vi "Dashboard Main.vi"() -> ()   [LabVIEW 2016]
uses:
  <vilib>/Utility/miscctls.llb/LVRowAndColumnTypeDef.ctl
  <vilib>/event_ctls.llb/eventvkey.ctl
  <vilib>/Rock Robotics/Network Tables/NT Read Numeric Array.vi
  <vilib>/Rock Robotics/Network Tables/NT Write Boolean.vi
  <vilib>/Rock Robotics/WPI/Dashboard/WPI_DashboardLogging Global.vi
panel:
  out "Background":bool
  in  "Camera Settings Right":T1={"Frame Rate"=30, "Compression"=30, "Size"=1, "DB Camera Config"=FALSE} {"Frame Rate" scale=1.0..30.0; "Compression" scale=100.0..-1.0; "Size" items=["640x480", "320x240", "160x120"]}
  in  "Camera Name Right":string(combo)="No Camera Selection"
  out "Camera Info":cluster{"Mbps LED":bool, "Mbps":dbl, "fps":dbl} {"fps" format="%#.1g"; "Mbps" format="%#.1g"}
  in  "Camera Settings":T1={"Frame Rate"=30, "Compression"=30, "Size"=1, "DB Camera Config"=FALSE} {"Frame Rate" scale=1.0..30.0; "Compression" scale=100.0..-1.0; "Size" items=["640x480", "320x240", "160x120"]}
  in  "TCP":refnum<k5>
  in  "Rec Mode":enum32{"Stop", "Record", "Playback"}(radio)
  out "Robot IP":string
  out "Image Message":string="Timeout in Camera Communications"
  in  "Dashboard Tab":T2(tab)
  in  "GoFast":bool
  in  "Select Auto":string(combo)="Select Autonomous ..."
  out "NT Connection":bool
  out "MotorChart R":cluster{"Numeric":dbl, "Numeric":dbl}(graph)
  out "MotorChart L":cluster{"Numeric":dbl, "Numeric":dbl}(graph)
  out "MotorSliders R":cluster{"MotorSlide1":dbl, "MotorSlide2":dbl} {"MotorSlide2" scale=-1.0..1.0 scale format="%#_2e"; "MotorSlide1" scale=-1.0..1.0 scale format="%#_2e"}
  out "MotorSliders L":cluster{"MotorSlide1":dbl, "MotorSlide2":dbl} {"MotorSlide2" scale=-1.0..1.0 scale format="%#_2e"; "MotorSlide1" scale=-1.0..1.0 scale format="%#_2e"}
  out "Gyro":dbl(knob) scale=0.0..360.0
  out "JS1 Z":dbl(slide) scale=-1.0..1.0 scale format="%#_2e"
  out "JS1 Graph":cluster{"X":dbl, "Y":dbl}[](graph)
  out "JS1 Buttons":T3
  out "JS2 Z":dbl(slide) scale=-1.0..1.0 scale format="%#_2e"
  out "JS2 Graph":cluster{"X":dbl, "Y":dbl}[](graph)
  out "JS2 Buttons":T3
  out "Mode":T4(ring)=enum."Auto Disabled"
  in  "Trim":dbl(slide)=0.5612244897959183 scale=0.0..1.0
  out "Sonar":dbl
  out "Camera Image Right":T5(plugin-control)
  in  "DB/String 9":string
  in  "DB/String 8":string
  in  "DB/String 7":string
  in  "DB/String 6":string
  in  "DB/String 5":string
  in  "DB/String 4":string
  in  "DB/String 3":string
  in  "DB/String 2":string
  in  "DB/String 1":string
  in  "DB/String 0":string
  in  "DB/Slider 0":dbl(slide) scale=0.0..1.0
  in  "DB/Slider 1":dbl(slide) scale=0.0..5.0
  in  "DB/Slider 2":dbl(slide)=11.111111111111112 caption="Autonomous Stop" scale=0.0..50.0
  in  "DB/Slider 3":dbl(slide)=0.6565656565656566 caption="Autonomous Trim" scale=0.0..1.0
  out "DB/LED 3":bool
  out "DB/LED 2":bool
  out "DB/LED 1":bool
  out "DB/LED 0":bool
  in  "DB/Button 3":bool
  in  "DB/Button 2":bool
  in  "DB/Button 1":bool
  in  "DB/Button 0":bool caption="New Name"
  in  "Scaling factor (V/in)":dbl=0.0098
  out "distance":dbl(slide)=125.0 scale=0.0..250.0 scale format="%3d"
  out "Z Acceleration":dbl
  out "Y Acceleration":dbl
  out "X Acceleration":dbl
  in  "Test Slider":dbl(slide) scale=0.0..100.0 scale format="%#_3g"
  in  "On/Off":bool caption="Solenoid"
  in  "Test Name":u16(ring) items=["Select the test to run..."]
  in  "Test Tree":string(tree)
  in  "Motor":cluster{"Value":dbl, "Enable":bool} {"Value" scale=-1.0..1.0 scale format="%#_3g"}
  out "Progress":T6 {"Test Progress" scale=0.0..100.0}
  in  "Rev/Fwd":cluster{"Forward":bool, "Reverse":bool}
  in  "Test Ring":u16(ring) items=["Monochrome", "Color"]
  out "Cmd Status":string
  in  "Execute Command":bool
  in  "Command Params":string[][](table)
  in  "Command Selection":i32(listbox)
  in  "CheckList":i32(listbox)
  out "Tree":string(tree)
  out "Camera Image":T5(plugin-control)
  in  "Camera Name":string(combo)="No Camera Selection"
  # "HW"
  # "HW"
  # "Joysticks"
  # "Drive Motors"
  # "Front"
  # "Right"
  # "Left"
  # "Back"
  # "This tab is a great place for autonomous settings and robot-specific values.\nPlace controls and indicators inside this tab and match name to\nDashboard Variables on robot. You can also delete this comment."
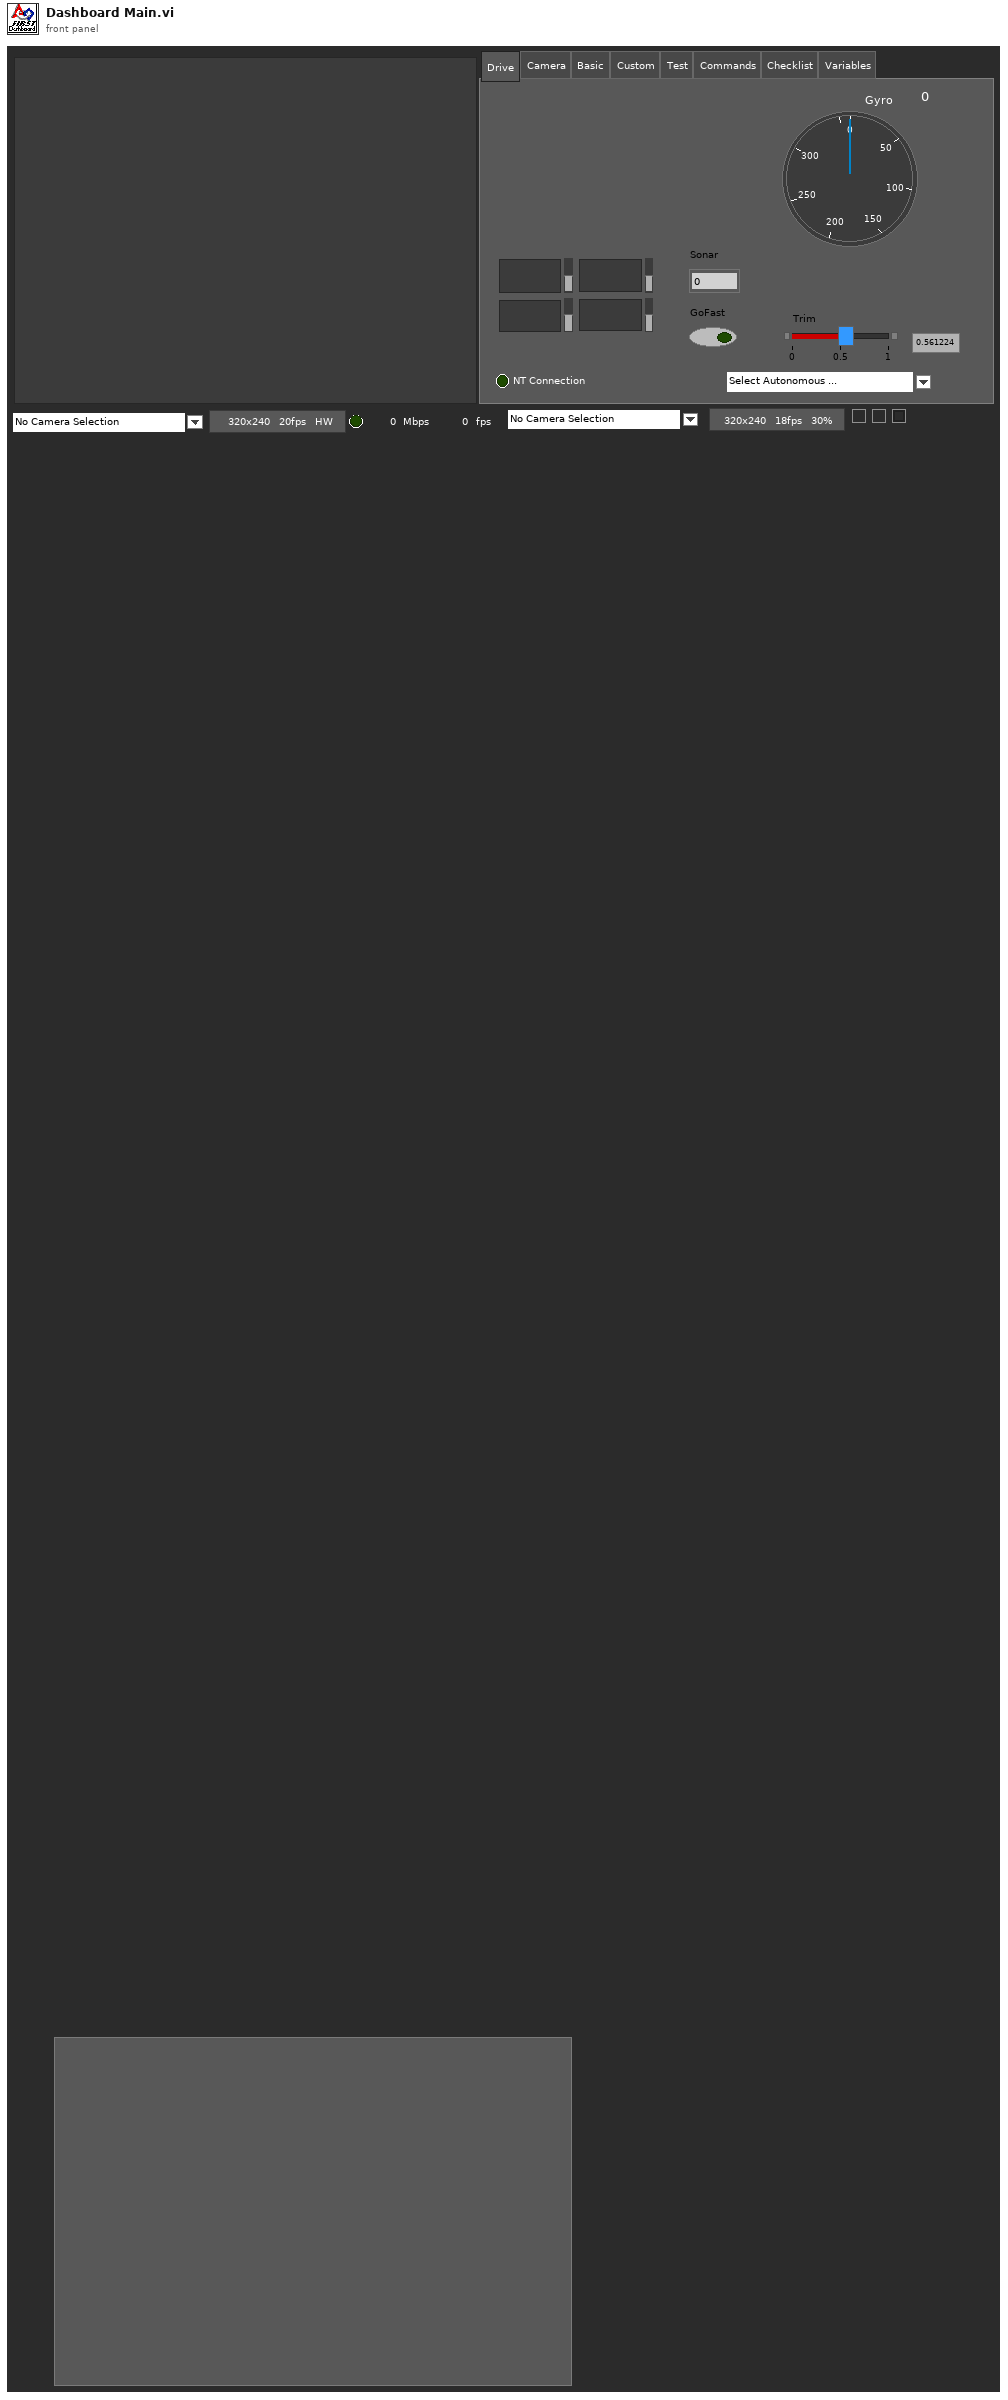
[diagram p1: front panel]
types:
  T1 = cluster{"Frame Rate":i32, "Compression":i32, "Size":u16, "DB Camera Config":bool}
  T2 = enum32{"Drive", "Camera", "Basic", "Custom", "Test", "Commands", "Checklist", "Variables"}
  T3 = cluster{bool, bool, bool, bool, bool, bool, bool, bool, bool, bool, bool, bool}
  T4 = enum8{"Tele-Op Disabled", "Tele-Op Enabled", "Auto Disabled", "Auto Enabled", "Test Disabled", "Test Enabled", "Disconnected", "No Code", "E-Stop"}
  T5 = typedef "IMAQ Image.ctl" = refnum<image>
  T6 = cluster{"Test Progress":u8, "Test Progress Text":string}
  T7 = typedef "Image Type" = u32
  T8 = cluster{"IDs":cluster{"RPC field ID":u16, "Unique ID":u16}, "String":string}
  T9 = enum32{"Drive", "Basic", "Custom", "Test", "Checklist", "Variables"}
  T10 = cluster{"Error Strings":string, "Disable Counts":cluster{u16, u16}, "Rail Faults":cluster{u16, u16, u16}, "Robot IP":string, "DB Mode":u8, "Event Info":cluster{"Name":string, "Type":u8, "Number":u16, "Replay":u8}}
  T11 = cluster{"Storage":cluster{"Disk Free":u64, "RAM Block":u32, "RAM free":u32}, "CPU Utilization":cluster{"CPU % ISR":sgl, "CPU % Time Crit":sgl, "CPU % Timed Str":sgl, "CPU % High":sgl, "CPU % Above":sgl, "CPU % Normal":sgl, "CPU % Low":sgl}, "CAN":cluster{"% Bus Utilization":sgl, "Bus Off Cnt":u32, "TX_FIFO Full Cnt":u32, "Receive Error Cnt":u8, "Transmit Error Cnt":u8}, "HID":cluster{"HID Outputs":u32, "Rumble Low":u16, "Rumble High":u16}[]}
  T12 = cluster{"Status bits":cluster{"Test Mode":bool, "Autonomous":bool, "Enabled":bool, "Code Start":bool, "Brownout":bool, "Reserved 2":bool, "Reserved 3":bool, "E-Stop":bool}, "Code Trace":cluster{"Disabled":bool, "TeleOp":bool, "Auto":bool, "Test":bool}, "Controller Type":enum16{"unknown", "cRIO", "roboRio"}, "Code?":enum16{"unknown", "noCode", "code"}, "Battery V":dbl}
  T13 = cluster{"Control Bits":cluster{"TestMode":bool, "Autonomous":bool, "Enabled":bool, "FMS Present":bool, bool, bool, bool, "E-Stop":bool}, "Team Station ":u8, "Countdown":sgl, "Joystick Values":cluster{"Axes":dbl[], "Buttons":bool[], "POVs":i16[]}[]}
  T14 = cluster{"Axes":dbl[], "Buttons":bool[], "POVs":i16[]}[]
  T15 = cluster{"Axes":dbl[], "Buttons":bool[], "POVs":i16[]}
  T16 = cluster{"Buttons[0]":bool, "Buttons[1]":bool, "Buttons[2]":bool, "Buttons[3]":bool, "Buttons[4]":bool, "Buttons[5]":bool, "Buttons[6]":bool, "Buttons[7]":bool, "Buttons[8]":bool, "Buttons[9]":bool, "Buttons[10]":bool, "Buttons[11]":bool}
  T17 = cluster{"Camera Image":refnum<vi>, "Dashboard Tab":refnum<vi>, "Background":refnum<vi>, "Rec Mode":refnum<vi>, "Test Slider":refnum<vi>, "On/Off ":refnum<vi>, "Test Ring":refnum<vi>, "Rev/Fwd":refnum<vi>, "Test Name":refnum<vi>, "Motor":refnum<vi>, "Progress":refnum<vi>, "CheckList":refnum<vi>, "Tree":refnum<vi>, "Test Tree":refnum<vi>, "Command Params":refnum<vi>, "Command Selection":refnum<vi>, "Execute Command":refnum<vi>, "Cmd Status":refnum<vi>, "Camera Settings":refnum<vi>, "Camera Name":refnum<vi>, "Camera Info":refnum<vi>, "Camera Settings Right":refnum<vi>, "Camera Name Right":refnum<vi>, "Camera Image Right":refnum<vi>}
  T18 = cluster{"Operation":enum16{"Update", "Clear"}, "Color Box":u32}[]
  T19 = typedef "eventvkey.ctl" = enum16{"ASCII", "Enter", "Return", "Shift", "Ctrl", "Alt", "Cmd", "Opt", "Caps", "NumLock", "Clear", "Break", "Up", "Down", "Left", "Right", "Insert", "Delete", "Home", "End", "PageUp", "PageDown", "Escape", "Help", "Pause", "ScrollLock", "F1", "F2", "F3", "F4", "F5", "F6", "F7", "F8", "F9", "F10", "F11", "F12", "F13", "F14", "F15", "F16", "F17", "F18", "F19", "F20", "F21", "F22", "F23", "F24", "Play", "VolumeUp", "VolumeDown", "Mute", "Two Byte Char"}
  T20 = cluster{"Image Size":bool, "Image Type":bool, "Pixel Value":bool, "ROI Information":bool, "Zoom Factor":bool}
  T21 = cluster{"Operation":enum16{"Update", "Clear"}, "Color Box":u32}
  T22 = typedef "LVRowAndColumnTypeDef.ctl" = cluster{"Row":i32, "Column":i32}
  T23 = cluster{"Shift":bool, "Ctrl":bool, "Alt":bool, "Cmd":bool, "Opt":bool}
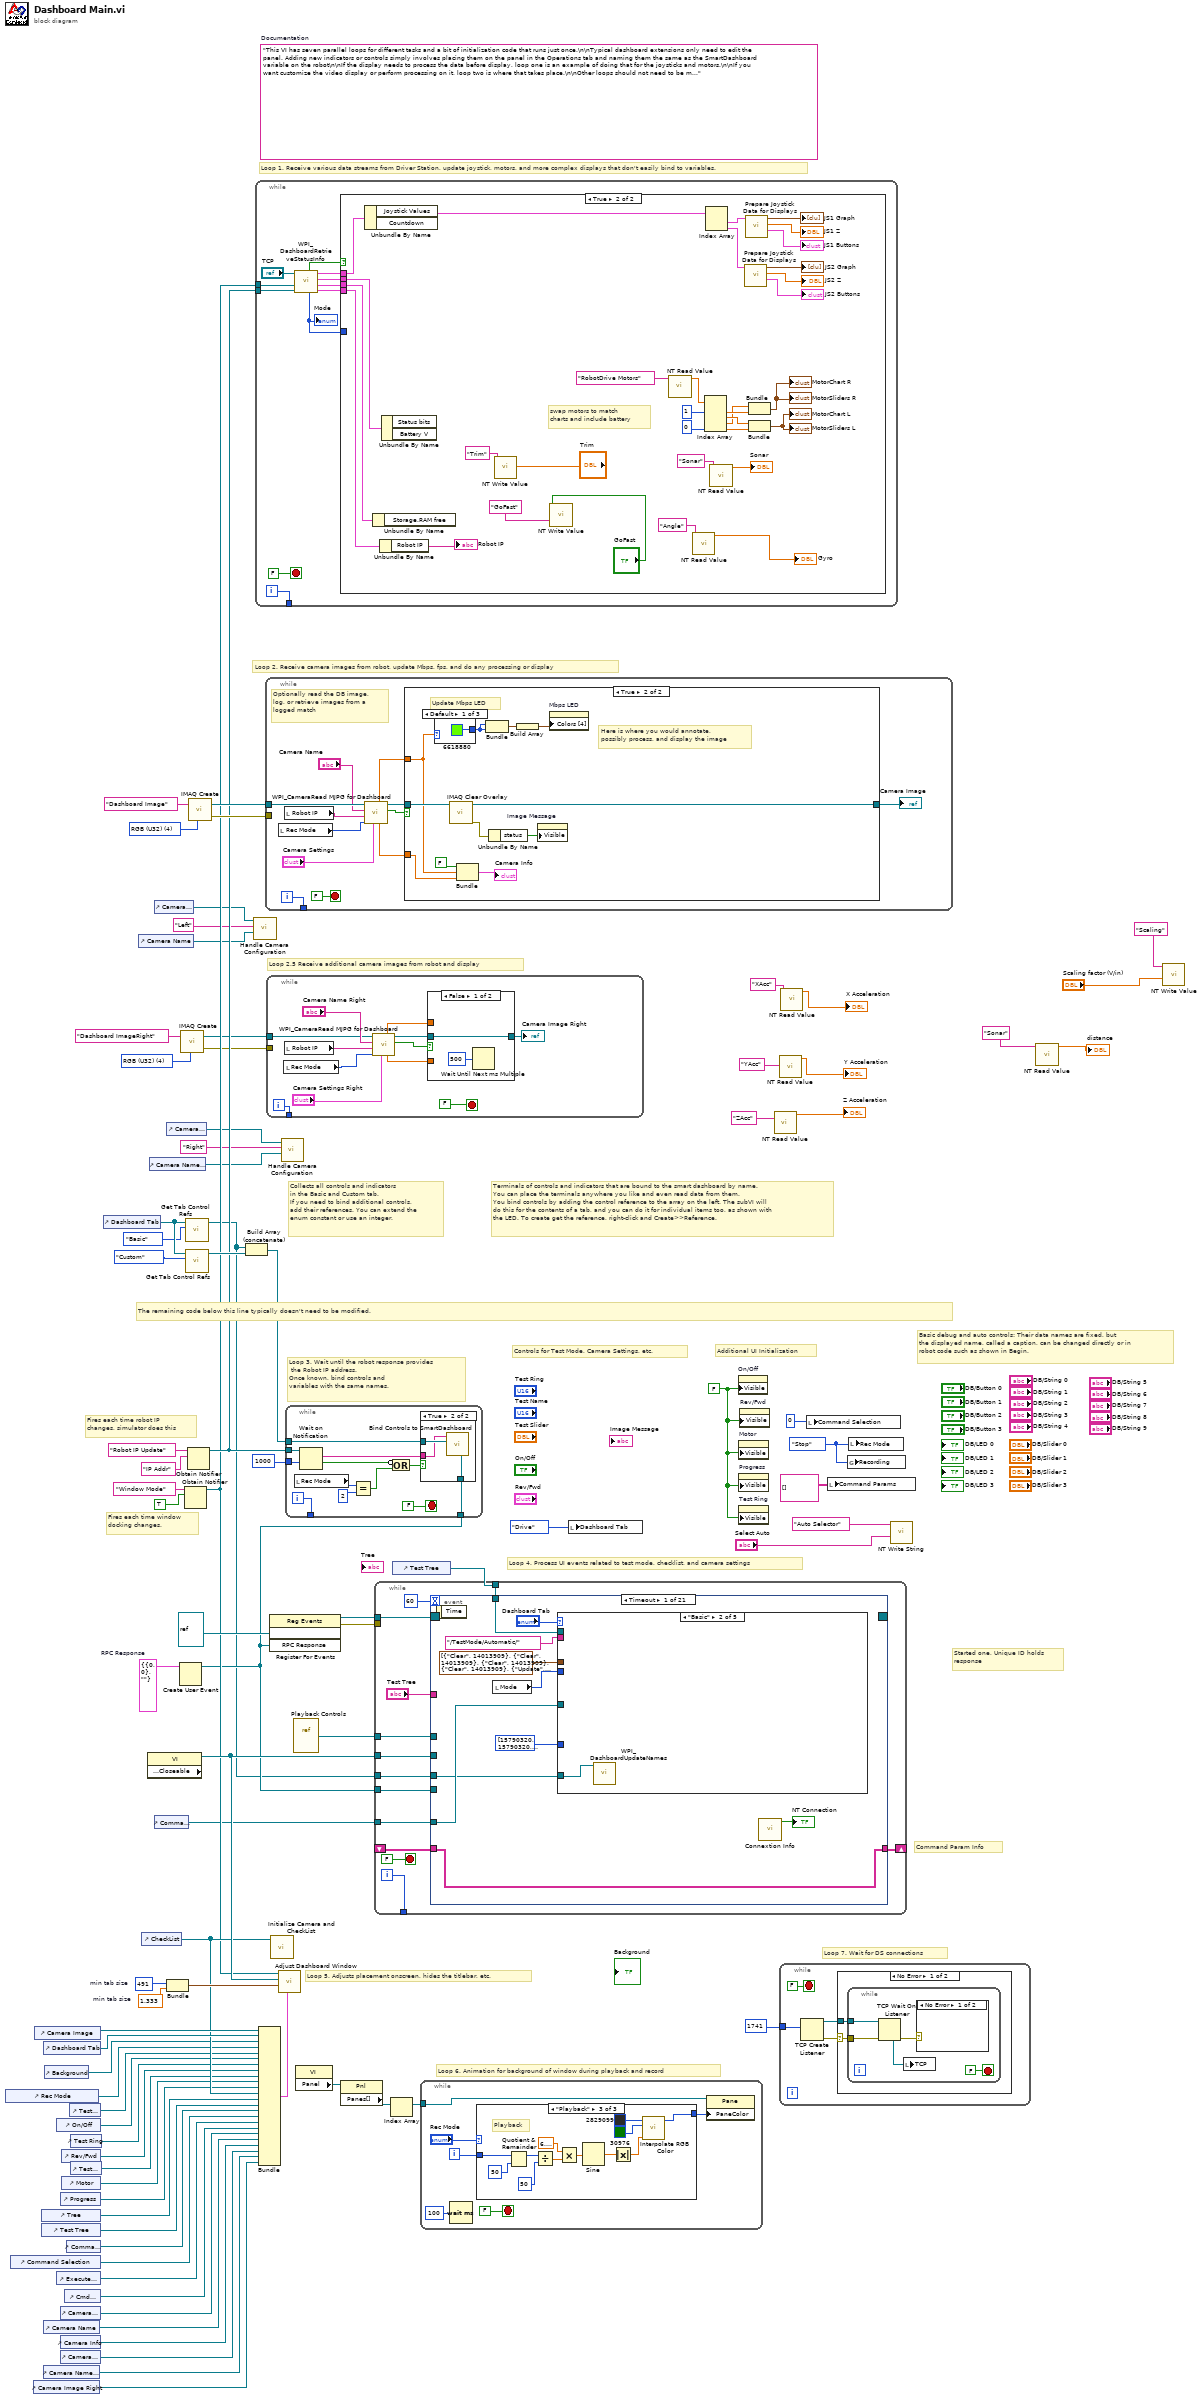
[diagram p0: block diagram]
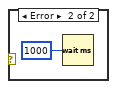
[diagram p3: hidden frame]
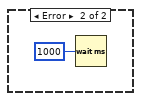
[diagram p4: hidden frame]
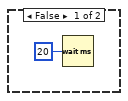
[diagram p5: hidden frame]
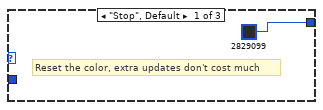
[diagram p6: hidden frame]
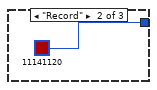
[diagram p7: hidden frame]
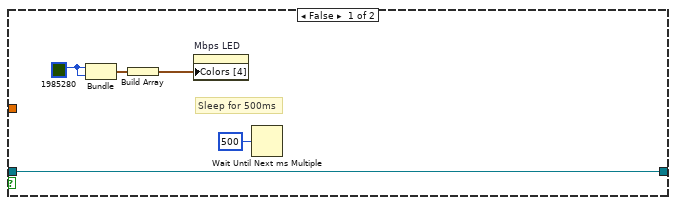
[diagram p9: hidden frame]
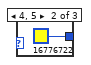
[diagram p10: hidden frame]
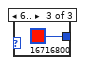
[diagram p11: hidden frame]
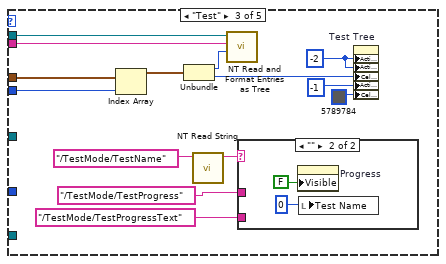
[diagram p13: hidden frame]
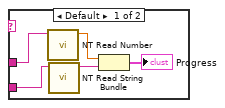
[diagram p14: hidden frame]
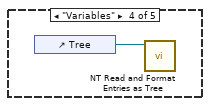
[diagram p15: hidden frame]
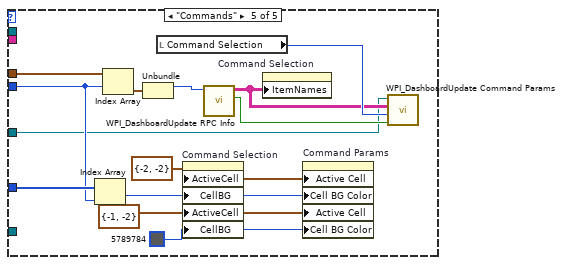
[diagram p16: hidden frame]
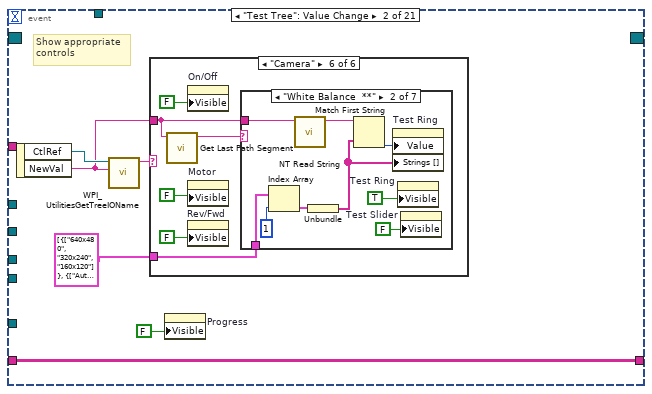
[diagram p17: hidden frame]
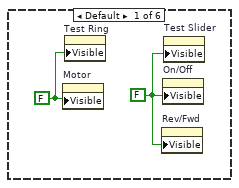
[diagram p18: hidden frame]
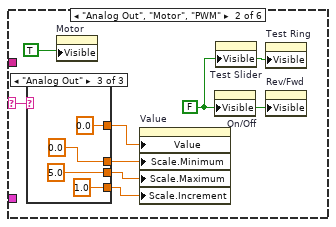
[diagram p19: hidden frame]
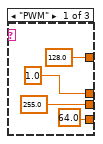
[diagram p20: hidden frame]
diagram:
  w22 = T7 4 items=["Grayscale (U8)", "Grayscale (I16)", "Grayscale (SGL)", "Complex (CSG)", "RGB (U32)", "HSL (U32)", "RGB (U64)"] ("Image Type")
  w38 = T8 {"IDs"={"RPC field ID"=0, "Unique ID"=0}, "String"=""}  # RPC Response
  w61 = 491  # min tab size
  w60 = 1.333  # min tab size
  w68 = enum32{"Stop", "Record", "Playback"}."Stop" ("Rec Mode")
  w45 = FALSE ("Visible")
  (unwired) "This VI has seven parallel loops for different tasks and a bit of initialization code that runs just once.\n\nTypical dashboard extensions only need to edit the panel. Adding new indicators or controls simply involves placing them on the panel in the Operations tab and naming them the same as the SmartDashboard variable on the robot\n\nIf the display needs to process the data before display, loop one is an example of doing that for the joysticks and motors.\n\nIf you want customize the video display or perform processing on it, loop two is where that takes place.\n\nOther loops should not need to be modified. They are pretty standard, and document the task they perform."  # Documentation
  w85 = T7 4 items=["Grayscale (U8)", "Grayscale (I16)", "Grayscale (SGL)", "Complex (CSG)", "RGB (U32)", "HSL (U32)", "RGB (U64)"] ("Image Type")
  # "Loop 2.5 Receive additional camera images from robot and display"
  # "Command Param Info"
  # "Started one, Unique ID holds\nresponse"
  # "Loop 7. Wait for DS connections"
  # "Basic debug and auto controls: Their data names are fixed, but\nthe displayed name, called a caption, can be changed directly or in\nrobot code such as shown in Begin."
  # "Controls for Test Mode, Camera Settings, etc."
  # "Additional UI Initialization"
  # "Loop 6. Animation for background of window during playback and record"
  # "Fires each time robot IP\nchanges, simulator does this"
  # "Fires each time window\ndocking changes."
  # "Collects all controls and indicators\nin the Basic and Custom tab.\nIf you need to bind additional controls,\nadd their references. You can extend the\nenum constant or use an integer."
  # "The remaining code below this line typically doesn't need to be modified."
  # "Loop 4. Process UI events related to test mode, checklist, and camera settings"
  # "Terminals of controls and indicators that are bound to the smart dashboard by name.\nYou can place the terminals anywhere you like and even read data from them.\nYou bind controls by adding the control reference to the array on the left. The subVI will\ndo this for the contents of a tab, and you can do it for individual items too, as shown with\nthe LED. To create get the reference, right-click and Create>>Reference."
  # "Loop 3. Wait until the robot response provides\n the Robot IP address.\nOnce known, bind controls and\nvariables with the same names."
  # "Loop 5. Adjusts placement onscreen, hides the titlebar, etc."
  # "Loop 1. Receive various data streams from Driver Station, update joystick, motors, and more complex displays that don't easily bind to variables."
  # "Loop 2. Receive camera images from robot, update Mbps, fps, and do any processing or display"
  n1 = control-ref of="Rec Mode"() -> (w51:refnum<vi>)
  n2 = control-ref of="Command Selection"() -> (w37:refnum<vi>)
  n3 = control-ref of="Camera Image Right"() -> (w13:refnum<vi>)
  n4 = control-ref of="Camera Image"() -> (w63:refnum<vi>)
  n5 = control-ref of="Tree"() -> (w55:refnum<vi>)
  n6 = control-ref of="Test Tree"() -> (w54:refnum<vi>)
  n7 = control-ref of="Dashboard Tab"() -> (w62:refnum<vi>)
  n8 = control-ref of="Camera Name"() -> (w28:refnum<vi>)
  n9 = control-ref of="Camera Name Right"() -> (w14:refnum<vi>)
  n10 = control-ref of="Background"() -> (w11:refnum<vi>)
  n11 = control-ref of="Execute Command"() -> (w39:refnum<vi>)
  n12 = control-ref of="On/Off"() -> (w49:refnum<vi>)
  n13 = control-ref of="Progress"() -> (w46:refnum<vi>)
  n14 = control-ref of="Camera Settings"() -> (w29:refnum<vi>)
  n15 = control-ref of="Camera Info"() -> (w27:refnum<vi>)
  n16 = control-ref of="Camera Settings Right"() -> (w15:refnum<vi>)
  n17 = control-ref of="Rev/Fwd"() -> (w47:refnum<vi>)
  n18 = control-ref of="Motor"() -> (w52:refnum<vi>)
  n19 = control-ref of="Cmd Status"() -> (w33:refnum<vi>)
  n20 = control-ref of="Command Params"() -> (w40:refnum<vi>)
  n21 = control-ref of="Test Slider"() -> (w50:refnum<vi>)
  n22 = control-ref of="Test Ring"() -> (w48:refnum<vi>)
  n23 = control-ref of="Test Name"() -> (w53:refnum<vi>)
  n24 = control-ref of="Dashboard Tab"() -> (w66:refnum<vi>)
  n25 = control-ref of="Camera Name"() -> (w30:refnum<vi>)
  n26 = control-ref of="CheckList"() -> (w56:refnum<vi>)
  n27 = property class="VI" props=["Front Panel.Closeable"]() -> (reference out=w67:refnum<vi>)  [unwired: 2 in, 2 out]
  n28 = control-ref of="Camera Name Right"() -> (w18:refnum<vi>)
  n29 = control-ref of="Camera Settings"() -> (w31:refnum<vi>)
  n30 = control-ref of="Command Params"() -> (w32:refnum<vi>)
  n31 = control-ref of="Camera Settings Right"() -> (w19:refnum<vi>)
  n32 = Bundle("min tab size"=w61, "min tab size"=w60) -> (w59:cluster{"min tab size":i32, "min tab size":dbl})  [unwired: 1 in]
  n33 = Create User Event(user event datatype=w38) -> (user event=w34:refnum<user-event>)  [unwired: 1 in, 1 out]
  n34 = call "IMAQ Create"("Image Name"="Dashboard ImageRight", "Image Type"=w22) -> ("New Image"=w21:T5, "error out"=w20:errorcluster)  [unwired: 2 in, 1 out]
  n35 = Obtain Notifier(name (unnamed)="Window Mode", notification data type=TRUE) -> (notifier out=w43:refnum<notifier>)  [unwired: 2 in, 2 out]
  n36 = call <vilib>:"Get Tab Control Refs.vi"("Page Index"=T9."Basic" ("Dashboard Tab"), "TabControl in"=w66) -> ("ControlsOnPage"=w26:refnum<vi>[])  [unwired: 9 in]
  n37 = call <vilib>:"Get Tab Control Refs.vi"("Page Index"=T9."Custom" ("Dashboard Tab"), "TabControl in"=w66) -> ("ControlsOnPage"=w65:refnum<vi>[])  [unwired: 9 in]
  n38 = Obtain Notifier(name (unnamed)="Robot IP Update", notification data type="IP Addr" ("name (unnamed)")) -> (notifier out=w44:refnum<notifier>)  [unwired: 2 in, 2 out]
  n39 = call "IMAQ Create"("Image Name"="Dashboard Image", "Image Type"=w85) -> ("New Image"=w83:T5, "error out"=w82:errorcluster)  [unwired: 2 in, 1 out]
  n40 = Build Array (concatenate)(w26, w65) -> (w64:refnum<vi>[])
  n41 = call "Handle Camera Configuration.vi"("CameraNameRef"=w30, "Camera File Name"="Left", "ClusterRef"=w31) -> ()  [unwired: 9 in]
  n42 = while {
    tunnel: [w95] -> _
    tunnel: w44 -> [w89]
    tunnel: w43 -> [w86]
    i -> [w95]
    stop <- FALSE stop-if-true
    n43 = call <vilib>:"WPI_DashboardRetrieveStatusInfo.vi"("Binding Refnum"=w89, "Window Mode Notifier"=w86, "TCP Cnx"="TCP") -> ("Power and Errors"=w90:T10, "Robot Metrics"=w93:T11, "Status Info"=w94:T12, "Control Info"=w91:T13, "Robot Mode"=w88:T4, "Process?"=w92:bool)  [unwired: 3 in]
    "Mode" <- w88
    n44 = case shown="True" w92 {
      tunnel: w94 -> [_ w129]
      tunnel: w93 -> [_ w128]
      tunnel: w91 -> [_ w127]
      tunnel: w90 -> [_ w126]
      tunnel: w88 -> [_ _]
      frame False {
        n45 = Wait (ms)(milliseconds to wait=u32 20) -> ()  [unwired: 1 out]
      }
      frame True {
        # "swap motors to match\ncharts and include battery"
        n46 = Unbundle By Name(w127) -> ("Joystick Values"=w117:T14)  [unwired: 1 out]
        n47 = Unbundle By Name(w128) -> ()  [unwired: 1 out]
        n48 = Unbundle By Name(w126) -> ("Robot IP"=→"Robot IP":string)
        n49 = Unbundle By Name(w129) -> ()  [unwired: 2 out]
        n50 = call-poly <vilib>:"NT Write Value.vi"("Numeric"="Trim", "Name"="Trim") -> ()  [unwired: 9 in, 1 out]
        n51 = call-poly <vilib>:"NT Write Value.vi"("Boolean"="GoFast", "Name"="GoFast") -> ()  [unwired: 9 in, 1 out]
        n52 = call-poly <vilib>:"NT Read Value.vi"("Name"="RobotDrive Motors") -> ("Numeric Array"=w107:dbl[])  [unwired: 9 in, 1 out]
        n53 = call-poly <vilib>:"NT Read Value.vi"("Name"="Angle") -> ("Numeric"=→"Gyro":dbl)  [unwired: 9 in, 1 out]
        n54 = Index Array(array=w107, index #1=1, index #4=0) -> (element #1=w121:dbl, element #2=w122:dbl, element #3=w120:dbl, element #4=w125:dbl)  [unwired: 2 in]
        n55 = Index Array(array=w117) -> (element #1=w116:T15, element #2=w112:T15)  [unwired: 2 in]
        n56 = call-poly <vilib>:"NT Read Value.vi"("Name"="Sonar") -> ("Numeric"=→"Sonar":dbl)  [unwired: 9 in, 1 out]
        n57 = call "Prepare Joystick Data for Displays.vi"("Joystick Values"=w112) -> ("Buttons"=→"JS2 Buttons":T16, "Z Axis"=→"JS2 Z":dbl, "Cartesian Data"=→"JS2 Graph":cluster{"X axis":dbl, "X axis":dbl}[])  [unwired: 8 in]
        n58 = call "Prepare Joystick Data for Displays.vi"("Joystick Values"=w116) -> ("Buttons"=→"JS1 Buttons":T16, "Z Axis"=→"JS1 Z":dbl, "Cartesian Data"=→"JS1 Graph":cluster{"X axis":dbl, "X axis":dbl}[])  [unwired: 8 in]
        n59 = Bundle("Numeric"=w120, "Numeric"=w121) -> (→"MotorChart R" →"MotorSliders R":cluster{"Numeric":dbl, "Numeric":dbl})  [unwired: 1 in]
        n60 = Bundle("Numeric"=w122, "Numeric"=w125) -> (→"MotorChart L" →"MotorSliders L":cluster{"Numeric":dbl, "Numeric":dbl})  [unwired: 1 in]
      }
    }
  }
  n61 = Bundle("Camera Image"=w63, "Dashboard Tab"=w62, "Background"=w11, "Rec Mode"=w51, "Test Slider"=w50, "On/Off"=w49, "Test Ring"=w48, "Rev/Fwd"=w47, "Test Name"=w53, "Motor"=w52, "Progress"=w46, "CheckList"=w56, "Tree"=w55, "Test Tree"=w54, "Command Params"=w40, "Command Selection"=w37, "Execute Command"=w39, "Cmd Status"=w33, "Camera Settings"=w29, "Camera Name"=w28, "Camera Info"=w27, "Camera Settings Right"=w15, "Camera Name Right"=w14, "Camera Image Right"=w13) -> (w12:T17)  [unwired: 1 in]
  n62 = while {
    tunnel: w83 -> [w139]
    tunnel: w82 -> [_]
    tunnel: [w140] -> _
    i -> [w140]
    stop <- FALSE stop-if-true
    # "Optionally read the DB image,\nlog, or retrieve images from a\nlogged match"
    n63 = local read "Rec Mode"() -> (w135:enum32{"Stop", "Record", "Playback"})
    n64 = local read "Robot IP"() -> (w134:string)
    n65 = call <vilib>:"WPI_CameraRead MJPG for Dashboard.vi"("Camera Settings"="Camera Settings", "Rec Mode"=w135, "Robot IP"=w134, "Camera Name"="Camera Name", "Refnum in"=w139) -> ("Active"=w137:bool, "Refnum out"=w138:T5, "FPS"=w136:dbl, "Bandwidth (Mbps)"=w133:dbl)  [unwired: 3 in]
    n66 = case shown="True" w137 {
      tunnel: w138 -> [w142 w153]
      tunnel: w133 -> [_ w150]
      tunnel: w136 -> [_ w151]
      tunnel: [w142 w147] -> w130
      frame False {
        w144 = u32 1985280 ("Color Box")
        # "Sleep for 500ms"
        n67 = Bundle("Color Box"=w144, "Color Box"=w144) -> (w145:cluster{"Color Box":u32, "Color Box":u32})  [unwired: 1 out]
        n68 = Build Array(w145) -> (w143:cluster{"Color Box":u32, "Color Box":u32}[])
        n69 = property on="Mbps LED" class="Bool (strict)"("Colors [4]"=w143) -> ()  [unwired: 2 in, 2 out]
        n70 = Wait Until Next ms Multiple(millisecond multiple=u32 500) -> ()  [unwired: 1 out]
      }
      frame True {
        # "Here is where you would annotate,\npossibly process, and display the image"
        # "Update Mbps LED"
        n71 = case shown="Default" w150 {
          tunnel: [u32 6618880 ("Color Box") u32 16776722 ("Color Box") u32 16716800 ("Color Box")] -> w154
          frame Default {
          }
          frame 4, 5 {
          }
          frame 6.. {
          }
        }
        n72 = call "IMAQ Clear Overlay"("Image"=w153) -> ("error out"=w156:errorcluster, "Image Out"=w147:T5)  [unwired: 2 in, 7 out]
        n73 = Bundle(FALSE, "Bandwidth (Mbps)"=w150, "FPS"=w151) -> (→"Camera Info":cluster{bool, "Bandwidth (Mbps)":dbl, "FPS":dbl})  [unwired: 1 in]
        n74 = Bundle("Color Box"=w154, "Color Box"=w154) -> (w155:cluster{"Color Box":u32, "Color Box":u32})  [unwired: 1 out]
        n75 = Unbundle By Name(w156) -> ("status"=w157:bool)
        n76 = Build Array(w155) -> (w152:cluster{"Color Box":u32, "Color Box":u32}[])
        n77 = property on="Image Message" class="Str"("Visible"=w157) -> ()  [unwired: 2 in, 2 out]
        n78 = property on="Mbps LED" class="Bool (strict)"("Colors [4]"=w152) -> ()  [unwired: 2 in, 2 out]
      }
    }
    "Camera Image" <- w130
  }
  n79 = while {
    tunnel: w21 -> [w171]
    tunnel: w20 -> [_]
    tunnel: [w165] -> _
    i -> [w165]
    stop <- FALSE stop-if-true
    n80 = local read "Rec Mode"() -> (w169:enum32{"Stop", "Record", "Playback"})
    n81 = local read "Robot IP"() -> (w170:string)
    n82 = call <vilib>:"WPI_CameraRead MJPG for Dashboard.vi"("Camera Settings"="Camera Settings Right", "Rec Mode"=w169, "Robot IP"=w170, "Camera Name"="Camera Name Right", "Refnum in"=w171) -> ("Active"=w164:bool, "Refnum out"=w167:T5, "FPS"=w162:dbl, "Bandwidth (Mbps)"=w163:dbl)  [unwired: 3 in]
    n83 = case shown="False" w164 {
      tunnel: w167 -> [w173 w175]
      tunnel: w163 -> [_ _]
      tunnel: w162 -> [_ _]
      tunnel: [w173 w175] -> w161
      frame False {
        n84 = Wait Until Next ms Multiple(millisecond multiple=u32 500) -> ()  [unwired: 1 out]
      }
      frame True {
      }
    }
    "Camera Image Right" <- w161
  }
  n85 = register-events(refnum<vi> refnum, w34) -> (reference out=w72:refnum<event-registration>, error out=w71:errorcluster)  [unwired: 2 in]
  n86 = call "Initialize Camera and CheckList.vi"("ListBox in"=w56) -> ()  [unwired: 11 in]
  n87 = call "Adjust Dashboard Window.vi"("Sizing Refnums"=w12, "Size Constraints"=w59, "VI"=w67, "WIn Mode"=w43) -> ()  [unwired: 8 in]
  n88 = call "Handle Camera Configuration.vi"("CameraNameRef"=w18, "Camera File Name"="Right", "ClusterRef"=w19) -> ()  [unwired: 9 in]
  n89 = while {
    tunnel: w64 -> [w187]
    tunnel: w44 -> [w185]
    tunnel: [w183] -> _
    tunnel: u32 1000 ("milliseconds to wait") -> [w182]
    tunnel: w34 -> [w176]
    i -> [w183]
    stop <- FALSE stop-if-true
    n90 = local read "Rec Mode"() -> (w178:enum32{"Stop", "Record", "Playback"})
    n91 = Wait on Notification(notifier=w185, timeout in ms (-1)=w182) -> (notification=w184:string, timed out?=w180:bool)  [unwired: 2 in, 2 out]
    n92 = Equal?(x=w178, y=u16 2 ("Rec Mode")) -> (x = y?=w179:bool)
    n93 = Compound Arithmetic op=OR(invert w180, w179) -> (w181:bool)
    n94 = case shown="True" w181 {
      tunnel: w187 -> [_ w190]
      tunnel: w184 -> [_ w189]
      tunnel: w176 -> [_ w188]
      frame False {
      }
      frame True {
        n95 = call <vilib>:"Bind Controls to SmartDashboard.vi"("RPC ref"=w188, "Bound Control Refs"=w190, "Server IP Address"=w189) -> ()  [unwired: 9 in]
      }
    }
  }
  n96 = vi-ref "Playback Controls.vi"() -> (w73:refnum<vi>)
  n97 = property class="VI"() -> ("Panel"=w75:refnum<vi>)  [unwired: 2 in, 2 out]
  n98 = property class="Pnl"(reference=w75) -> ("Panes[]"=w76:refnum<vi>[])  [unwired: 1 in, 2 out]
  n99 = Index Array(array=w76) -> (element=w74:refnum<vi>)  [unwired: 1 in]
  n100 = control-ref of="Test Tree"() -> (w77:refnum<vi>)
  n101 = while {
    tunnel: [w200] -> _
    tunnel: w77 -> [w199]
    tunnel: w73 -> [w198]
    tunnel: w72 -> [w197]
    tunnel: w71 -> [_]
    tunnel: w67 -> [w196]
    tunnel: w34 -> [w195]
    tunnel: w32 -> [w194]
    shift-right: [w193] -> _
    shift-left: _ -> [w192]
    tunnel: w26 -> [w191]
    i -> [w200]
    stop <- FALSE stop-if-true
    n102 = event shown="[0] Timeout" {
      selector: w197 -> [_ _ _ _ _ _ _ _ _ _ _ _ _ _ _ _ _ _ _ _ _]
      dyn-events: [_ _ _ _ _ _ _ _ _ _ _ _ _ _ _ _ w456 _ _ _ _] -> _
      timeout: u32 60 ("milliseconds to wait") -> [_ _ _ _ _ _ _ _ _ _ _ _ _ _ _ _ _ _ _ _ _]
      tunnel: w199 -> [w212 _ _ _ _ _ _ _ _ _ _ _ _ _ _ _ _ _ _ _ _]
      tunnel: "Test Tree" -> [_ _ _ _ _ _ _ _ _ _ _ w423 w431 w433 w437 w445 _ _ _ _ _]
      tunnel: w198 -> [_ _ _ _ _ _ _ _ _ _ _ _ _ _ _ _ w458 _ w476 _ _]
      tunnel: w196 -> [_ _ _ _ _ _ _ _ _ _ _ _ _ _ _ _ w454 _ _ _ _]
      tunnel: w195 -> [_ _ _ _ _ _ _ _ _ _ _ _ _ _ _ _ w450 _ _ _ _]
      tunnel: w194 -> [w207 _ _ _ _ _ w374 _ _ _ _ _ _ _ _ _ _ _ _ _ _]
      tunnel: [w206 w251 w353 w358 w367 w371 w372 w381 w391 w398 w410 w422 w429 w432 w436 w444 w449 w471 w473 w477 w488] -> w193
      tunnel: w192 -> [w206 w251 w353 w358 w367 w371 w372 _ _ w398 w410 w422 w429 w432 w436 w444 w449 w471 w473 w477 w488]
      tunnel: w191 -> [w204 _ _ _ _ _ _ _ _ _ _ _ _ _ _ _ _ _ _ _ _]
      event Timeout {
        n103 = event-data() -> ()  [unwired: 1 in, 1 out]
        n104 = local read "Mode"() -> (w209:T4)
        n105 = case shown="\"Basic\"" "Dashboard Tab" {
          tunnel: w212 -> [_ _ w228 _ _]
          tunnel: "/TestMode/Automatic/" ("Name Pattern") -> [_ _ w227 _ _]
          tunnel: T18 [{"Operation"=enum."Clear", "Color Box"=14013909}, {"Operation"=enum."Clear", "Color Box"=14013909}, {"Operation"=enum."Clear", "Color Box"=14013909}, {"Operation"=enum."Clear", "Color Box"=14013909}, {"Operation"=enum."Update", "Color Box"=14013909}, {"Operation"=enum."Update", "Color Box"=16777215}, {"Operation"=enum."Clear", "Color Box"=14013909}, {"Operation"=enum."Clear", "Color Box"=14013909}, {"Operation"=enum."Clear", "Color Box"=14013909}] -> [_ _ w220 _ w244]
          tunnel: w209 -> [_ _ w219 _ w243]
          tunnel: u32[] [15790320, 15790320, 15790320, 15790320, 16777215, 16777215, 15790320, 15790320, 15790320] -> [_ _ _ _ w249]
          tunnel: w207 -> [_ _ _ _ w237]
          tunnel: w204 -> [_ w214 _ _ _]
          frame "Custom", Default {
          }
          frame "Basic" {
            n106 = call <vilib>:"WPI_DashboardUpdateNames.vi"("Controls on Tab"=w214) -> ()  [unwired: 11 in]
          }
          frame "Test" {
            w226 = -2 ("Active Item:Row Number")
            n107 = Index Array(array=w220, index=w219) -> (element=w221:T21)
            n108 = Unbundle(w221) -> ("Operation"=w222:enum16{"Update", "Clear"}, "Color Box"=w223:u32)
            n109 = call <vilib>:"NT Read String.vi"("Name"="/TestMode/TestName") -> ("String"=w217:string)  [unwired: 9 in, 1 out]
            n110 = call <vilib>:"NT Read and Format Entries as Tree.vi"("Operation"=w222, "Name Pattern"=w227, "Tree Refnum"=w228) -> ()  [unwired: 7 in, 2 out]
            n111 = case shown="\"\"" w217 {
              tunnel: "/TestMode/TestProgress" ("Name") -> [w230 _]
              tunnel: "/TestMode/TestProgressText" ("Name") -> [w229 _]
              frame Default {
                n112 = call <vilib>:"NT Read Number.vi"("Name"=w230) -> ("Numeric"=w231:dbl)  [unwired: 9 in, 1 out]
                n113 = call <vilib>:"NT Read String.vi"("Name"=w229) -> ("String"=w232:string)  [unwired: 9 in, 1 out]
                n114 = Bundle("Numeric"=w231, "String"=w232) -> (→"Progress":cluster{"Numeric":dbl, "String":string})  [unwired: 1 in]
              }
              frame "" {
                n115 = property on="Progress" class="Clust (strict)"("Visible"=FALSE) -> ()  [unwired: 2 in, 2 out]
                n116 = local write "Test Name"(u16 0) -> ()
              }
            }
            n117 = property on="Test Tree" class="Tree (strict)"("Active Item Row Number"=w226, "ActiveColNum"=w226, "CellBG"=w223, "Active Item Row Number"=-1 ("Active Item:Row Number"), "CellBG"=u32 5789784 ("Color Box")) -> ()  [unwired: 2 in, 2 out]
          }
          frame "Variables" {
            n118 = control-ref of="Tree"() -> (w236:refnum<vi>)
            n119 = call <vilib>:"NT Read and Format Entries as Tree.vi"("Tree Refnum"=w236) -> ()  [unwired: 9 in, 2 out]
          }
          frame "Commands" {
            w245 = u32 5789784 ("Color Box")
            w246 = T22 {"Row"=-1, "Column"=-2} ("Active Cell:Active Cell")
            w248 = T22 {"Row"=-2, "Column"=-2} ("Active Cell:Active Cell")
            n120 = Index Array(array=w249, index=w243) -> (element=w247:u32)
            n121 = Index Array(array=w244, index=w243) -> (element=w242:T21)
            n122 = Unbundle(w242) -> ("Operation"=w241:enum16{"Update", "Clear"})  [unwired: 1 out]
            n123 = local read "Command Selection"() -> (w240:i32)
            n124 = property on="Command Selection" class="MCListbox (strict)"("ActiveCell"=w248, "CellBG"=w247, "ActiveCell"=w246, "CellBG"=w245) -> ()  [unwired: 2 in, 2 out]
            n125 = call <vilib>:"WPI_DashboardUpdate RPC Info.vi"("Operation"=w241) -> ("update"=w239:bool, "commands"=w238:string[][])  [unwired: 9 in]
            n126 = property on="Command Selection" class="MCListbox (strict)"("ItemNames"=w238) -> ()  [unwired: 2 in, 2 out]
            n127 = property on="Command Params" class="Tbl (strict)"("Active Cell"=w248, "Cell BG Color"=w247, "Active Cell"=w246, "Cell BG Color"=w245) -> ()  [unwired: 2 in, 2 out]
            n128 = call <vilib>:"WPI_DashboardUpdate Command Params.vi"("Update"=w239, "NewVal"=w240, "Commands"=w238, "Param Tbl"=w237) -> ()  [unwired: 7 in, 1 out]
          }
        }
        n129 = call <vilib>:"Connextion Info.vi"() -> ("Connected"=→"NT Connection":bool)  [unwired: 10 in, 1 out]
      }
      event "Test Tree": Value Change {
        # "Show appropriate\ncontrols"
        n130 = event-data() -> ("CtlRef"=w254:refnum<vi>, "NewVal"=w252:string)  [unwired: 1 in]
        n131 = call <vilib>:"WPI_UtilitiesGetTreeIOName.vi"("NewVal"=w252, "TreeControl in"=w254) -> ("I/O Name"=w255:string)  [unwired: 9 in]
        n132 = case shown="\"Camera\"" w255 {
          selector: w255 -> [_ w262 _ w284 w293 _]
          tunnel: w252 -> [_ _ w281 w283 _ w300]
          tunnel: cluster{string[]}[] [{["640x480", "320x240", "160x120"]}, {["Auto", "Fixed indoor", "Fixed outdoor 1", "Fixed outdoor 2", "Fixed fluorescent 1", "Fixed fluorescent 2", "Hold current"]}, {["Auto", "Flicker-free 50 Hz", "Flicker-free 60 Hz", "Hold current"]}, {["None", "Prioritize frame rate", "Prioritize image quality"]}, {["Monochrome", "Color"]}] -> [_ _ _ _ _ w299]
          frame Default {
            w257 = FALSE ("Visible")
            w256 = FALSE ("Visible")
            n133 = property on="Motor" class="Clust (strict)"("Visible"=w256) -> ()  [unwired: 2 in, 2 out]
            n134 = property on="Test Ring" class="Ring (strict)"("Visible"=w256) -> ()  [unwired: 2 in, 2 out]
            n135 = property on="Rev/Fwd" class="Clust (strict)"("Visible"=w257) -> ()  [unwired: 2 in, 2 out]
            n136 = property on="On/Off" class="Bool (strict)"("Visible"=w257) -> ()  [unwired: 2 in, 2 out]
            n137 = property on="Test Slider" class="Slide (strict)"("Visible"=w257) -> ()  [unwired: 2 in, 2 out]
          }
          frame "Analog Out", "Motor", "PWM" {
            w263 = FALSE ("Visible")
            n138 = case shown="\"Analog Out\"" w262 {
              tunnel: [1.0 ("Value") -1.0 ("Value") 0.0 ("Value")] -> w261
              tunnel: [255.0 ("Value") 1.0 ("Value") 5.0 ("Value")] -> w260
              tunnel: [128.0 ("Value") 0.0 ("Value") 0.0 ("Value")] -> w259
              tunnel: [64.0 ("Value") 0.5 ("Value") 1.0 ("Value")] -> w258
              frame "PWM" {
              }
              frame "Motor", Default {
              }
              frame "Analog Out" {
              }
            }
            n139 = property on="Motor" class="Clust (strict)"("Visible"=TRUE) -> ()  [unwired: 2 in, 2 out]
            n140 = property on="Value" class="Slide (strict)"("Value"=w259, "Scale.Minimum"=w261, "Scale.Maximum"=w260, "Scale.Increment"=w258) -> ()  [unwired: 2 in, 2 out]
            n141 = property on="On/Off" class="Bool (strict)"("Visible"=w263) -> ()  [unwired: 2 in, 2 out]
            n142 = property on="Test Slider" class="Slide (strict)"("Visible"=w263) -> ()  [unwired: 2 in, 2 out]
            n143 = property on="Test Ring" class="Ring (strict)"("Visible"=w263) -> ()  [unwired: 2 in, 2 out]
            n144 = property on="Rev/Fwd" class="Clust (strict)"("Visible"=w263) -> ()  [unwired: 2 in, 2 out]
          }
          frame "Servo" {
            w279 = FALSE ("Visible")
            n145 = call <vilib>:"NT Read Number.vi"("Name"=w281) -> ("Numeric"=w280:dbl)  [unwired: 9 in, 1 out]
            n146 = property on="Test Slider" class="Slide (strict)"("Visible"=TRUE, "Scale.Maximum"=170.0 ("Scale.Range:Maximum")) -> ()  [unwired: 2 in, 2 out]
            n147 = local write "Test Slider"(w280) -> ()
            n148 = property on="Motor" class="Clust (strict)"("Visible"=w279) -> ()  [unwired: 2 in, 2 out]
            n149 = property on="Rev/Fwd" class="Clust (strict)"("Visible"=w279) -> ()  [unwired: 2 in, 2 out]
            n150 = property on="On/Off" class="Bool (strict)"("Visible"=w279) -> ()  [unwired: 2 in, 2 out]
            n151 = property on="Test Ring" class="Ring (strict)"("Visible"=w279) -> ()  [unwired: 2 in, 2 out]
          }
          frame "Relay", "Solenoid" {
            w282 = FALSE ("Visible")
            n152 = property on="Motor" class="Clust (strict)"("Visible"=w282) -> ()  [unwired: 2 in, 2 out]
            n153 = property on="Test Slider" class="Slide (strict)"("Visible"=w282) -> ()  [unwired: 2 in, 2 out]
            n154 = Search and Replace String(input string=w283, search string="/Value  **", replace string="/Direction") -> (result string=w289:string)  [unwired: 5 in, 3 out]
            n155 = property on="Test Ring" class="Ring (strict)"("Visible"=w282) -> ()  [unwired: 2 in, 2 out]
            n156 = call <vilib>:"NT Read String.vi"("Name"=w289) -> ("String"=w287:string)  [unwired: 9 in, 1 out]
            n157 = Equal?(x="Both directions", y=w287) -> (x = y?=w285:bool)
            n158 = Not(x=w285) -> (.not. x?=w286:bool)
            n159 = property on="Rev/Fwd" class="Clust (strict)"("Visible"=w285) -> ()  [unwired: 2 in, 2 out]
            n160 = property on="On/Off" class="Bool (strict)"("Visible"=w286, "Caption.Text"=w284) -> ()  [unwired: 2 in, 2 out]
          }
          frame "Compressor", "Digital Out" {
            w292 = FALSE ("Visible")
            # "Get direction and finish"
            n161 = property on="Motor" class="Clust (strict)"("Visible"=w292) -> ()  [unwired: 2 in, 2 out]
            n162 = property on="Test Slider" class="Slide (strict)"("Visible"=w292) -> ()  [unwired: 2 in, 2 out]
            n163 = property on="Test Ring" class="Ring (strict)"("Visible"=w292) -> ()  [unwired: 2 in, 2 out]
            n164 = property on="On/Off" class="Bool (strict)"("Visible"=TRUE, "Caption.Text"=w293) -> ()  [unwired: 2 in, 2 out]
            n165 = property on="Rev/Fwd" class="Clust (strict)"("Visible"=FALSE) -> ()  [unwired: 2 in, 2 out]
          }
          frame "Camera" {
            n166 = call <vilib>:"Get Last Path Segment.vi"("String in"=w300) -> ("String out"=w301:string)  [unwired: 10 in]
            n167 = property on="On/Off" class="Bool (strict)"("Visible"=FALSE) -> ()  [unwired: 2 in, 2 out]
            n168 = property on="Motor" class="Clust (strict)"("Visible"=FALSE) -> ()  [unwired: 2 in, 2 out]
            n169 = property on="Rev/Fwd" class="Clust (strict)"("Visible"=FALSE) -> ()  [unwired: 2 in, 2 out]
            n170 = case shown="\"White Balance  **\"" w301 {
              tunnel: w300 -> [w307 w316 w325 w334 w343 _ w349]
              tunnel: w299 -> [w305 w313 w322 w331 w340 _ _]
              frame "Size  **" {
                n171 = Index Array(array=w305) -> (element=w304:cluster{string[]})  [unwired: 1 in]
                n172 = call <vilib>:"NT Read String.vi"("Name"=w307) -> ("String"=w306:string)  [unwired: 9 in, 1 out]
                n173 = Unbundle(w304) -> (w302:string[])
                n174 = Match First String(2:w302, 3:w306) -> (0:w303:i32)  [unwired: 1 out]
                n175 = property on="Test Ring" class="Ring (strict)"("Value"=w303, "Strings []"=w302) -> ()  [unwired: 2 in, 2 out]
                n176 = property on="Test Ring" class="Ring (strict)"("Visible"=TRUE) -> ()  [unwired: 2 in, 2 out]
                n177 = property on="Test Slider" class="Slide (strict)"("Visible"=FALSE) -> ()  [unwired: 2 in, 2 out]
              }
              frame "White Balance  **" {
                n178 = Index Array(array=w313, index=1) -> (element=w314:cluster{string[]})
                n179 = call <vilib>:"NT Read String.vi"("Name"=w316) -> ("String"=w315:string)  [unwired: 9 in, 1 out]
                n180 = Unbundle(w314) -> (w311:string[])
                n181 = Match First String(2:w311, 3:w315) -> (0:w310:i32)  [unwired: 1 out]
                n182 = property on="Test Ring" class="Ring (strict)"("Value"=w310, "Strings []"=w311) -> ()  [unwired: 2 in, 2 out]
                n183 = property on="Test Ring" class="Ring (strict)"("Visible"=TRUE) -> ()  [unwired: 2 in, 2 out]
                n184 = property on="Test Slider" class="Slide (strict)"("Visible"=FALSE) -> ()  [unwired: 2 in, 2 out]
              }
              frame "Exposure  **" {
                n185 = Index Array(array=w322, index=2) -> (element=w323:cluster{string[]})
                n186 = call <vilib>:"NT Read String.vi"("Name"=w325) -> ("String"=w324:string)  [unwired: 9 in, 1 out]
                n187 = Unbundle(w323) -> (w319:string[])
                n188 = Match First String(2:w319, 3:w324) -> (0:w320:i32)  [unwired: 1 out]
                n189 = property on="Test Ring" class="Ring (strict)"("Value"=w320, "Strings []"=w319) -> ()  [unwired: 2 in, 2 out]
                n190 = property on="Test Ring" class="Ring (strict)"("Visible"=TRUE) -> ()  [unwired: 2 in, 2 out]
                n191 = property on="Test Slider" class="Slide (strict)"("Visible"=FALSE) -> ()  [unwired: 2 in, 2 out]
              }
              frame "Exposure Priority  **" {
                n192 = Index Array(array=w331, index=3) -> (element=w332:cluster{string[]})
                n193 = call <vilib>:"NT Read String.vi"("Name"=w334) -> ("String"=w333:string)  [unwired: 9 in, 1 out]
                n194 = Unbundle(w332) -> (w328:string[])
                n195 = Match First String(2:w328, 3:w333) -> (0:w329:i32)  [unwired: 1 out]
                n196 = property on="Test Ring" class="Ring (strict)"("Value"=w329, "Strings []"=w328) -> ()  [unwired: 2 in, 2 out]
                n197 = property on="Test Ring" class="Ring (strict)"("Visible"=TRUE) -> ()  [unwired: 2 in, 2 out]
                n198 = property on="Test Slider" class="Slide (strict)"("Visible"=FALSE) -> ()  [unwired: 2 in, 2 out]
              }
              frame "Color Enable  **" {
                n199 = Index Array(array=w340, index=4) -> (element=w341:cluster{string[]})
                n200 = call <vilib>:"NT Read String.vi"("Name"=w343) -> ("String"=w342:string)  [unwired: 9 in, 1 out]
                n201 = Unbundle(w341) -> (w337:string[])
                n202 = Match First String(2:w337, 3:w342) -> (0:w338:i32)  [unwired: 1 out]
                n203 = property on="Test Ring" class="Ring (strict)"("Value"=w338, "Strings []"=w337) -> ()  [unwired: 2 in, 2 out]
                n204 = property on="Test Ring" class="Ring (strict)"("Visible"=TRUE) -> ()  [unwired: 2 in, 2 out]
                n205 = property on="Test Slider" class="Slide (strict)"("Visible"=FALSE) -> ()  [unwired: 2 in, 2 out]
              }
              frame Default {
                n206 = property on="Test Ring" class="Ring (strict)"("Visible"=FALSE) -> ()  [unwired: 2 in, 2 out]
                n207 = property on="Test Slider" class="Slide (strict)"("Visible"=FALSE) -> ()  [unwired: 2 in, 2 out]
              }
              frame "Brightness  **", "Color Level  **", "Compression  **", "FPS  **", "Sharpness  **" {
                n208 = call <vilib>:"NT Read Number.vi"("Name"=w349) -> ("Numeric"=w348:dbl)  [unwired: 9 in, 1 out]
                n209 = local write "Test Slider"(w348) -> ()
                n210 = property on="Test Slider" class="Slide (strict)"("Visible"=TRUE, "Scale.Maximum"=100.0 ("Scale.Range:Maximum")) -> ()  [unwired: 2 in, 2 out]
                n211 = property on="Test Ring" class="Ring (strict)"("Visible"=FALSE) -> ()  [unwired: 2 in, 2 out]
              }
            }
          }
        }
        n212 = property on="Progress" class="Clust (strict)"("Visible"=FALSE) -> ()  [unwired: 2 in, 2 out]
      }
      event "Test Name": Mouse Enter {
        # "Populate the ring with the list of tests"
        n213 = event-data() -> ()  [unwired: 1 in, 1 out]
        n214 = call <vilib>:"NT Read String Array.vi"("Name"="/TestMode/TestList") -> ("String Array"=w357:string[])  [unwired: 9 in, 1 out]
        n215 = Build Array (concatenate)("Select the test to run...", w357) -> (w356:string[])
        n216 = property on="Test Name" class="Ring (strict)"("Strings []"=w356) -> ()  [unwired: 2 in, 2 out]
      }
      event "Test Name": Value Change {
        w359 = FALSE ("Visible")
        # "Tell the robot the test name to run"
        n217 = event-data() -> ("NewVal"=w363:u16)  [unwired: 1 in]
        n218 = property on="Test Name" class="Ring (strict)"() -> ("Strings []"=w364:string[])  [unwired: 2 in, 2 out]
        n219 = local write "Progress"(T6 {"Test Progress"=0, "Test Progress Text"=""} ("Progress")) -> ()
        n220 = Index Array(array=w364, index=w363) -> (element=w362:string)
        n221 = call <vilib>:"NT Write String.vi"("String"=w362, "Name"="/TestMode/TestName") -> ()  [unwired: 9 in, 1 out]
        n222 = property on="Progress" class="Clust (strict)"("Visible"=TRUE) -> ()  [unwired: 2 in, 2 out]
        n223 = property on="Motor" class="Clust (strict)"("Visible"=w359) -> ()  [unwired: 2 in, 2 out]
        n224 = property on="Test Slider" class="Slide (strict)"("Visible"=w359) -> ()  [unwired: 2 in, 2 out]
        n225 = property on="On/Off" class="Bool (strict)"("Visible"=w359) -> ()  [unwired: 2 in, 2 out]
        n226 = property on="Rev/Fwd" class="Clust (strict)"("Visible"=w359) -> ()  [unwired: 2 in, 2 out]
        n227 = property on="Test Ring" class="Ring (strict)"("Visible"=w359) -> ()  [unwired: 2 in, 2 out]
      }
      event "Select Auto": Mouse Enter {
        # "Populate the combo box with the list of autonomous options"
        n228 = event-data() -> ()  [unwired: 1 in, 1 out]
        n229 = call <vilib>:"NT Read String Array.vi"("Name"="Auto List") -> ("String Array"=w366:string[])  [unwired: 9 in, 1 out]
        n230 = property on="Select Auto" class="CmbBox"("Strings[]"=w366) -> ()  [unwired: 2 in, 2 out]
      }
      event "Select Auto": Value Change {
        # "User modified the Auto Selection. Write to NT variable so robot knows."
        n231 = event-data() -> ("NewVal"=w369:string)  [unwired: 1 in]
        n232 = call <vilib>:"NT Write String.vi"("String"=w369, "Name"="Auto Selector") -> ()  [unwired: 9 in, 1 out]
      }
      event "Command Selection": Value Change {
        # "Get the params and show in table"
        n233 = event-data() -> ("NewVal"=w375:i32)  [unwired: 1 in]
        n234 = property on="Command Selection" class="MCListbox (strict)"() -> ("ItemNames"=w373:string[][])  [unwired: 2 in, 2 out]
        n235 = call <vilib>:"WPI_DashboardUpdate Command Params.vi"("NewVal"=w375, "Commands"=w373, "Param Tbl"=w374) -> ()  [unwired: 8 in, 1 out]
      }
      event "Execute Command": Value Change {
        # "Started one, Unique ID holds\nresponse"
        n236 = event-data() -> ()  [unwired: 1 in, 1 out]
        n237 = property on="Command Selection" class="MCListbox (strict)"() -> ("ItemNames"=w386:string[][])  [unwired: 2 in, 2 out]
        n238 = Index Array(array=w386, index (row)="Command Selection", index (col)=0) -> (element=w384:string)
        n239 = call <vilib>:"Invoke Commands.vi"("Command Params"="Command Params", "Function Name"=w384) -> ("Params"=w380:u8, "Started"=w379:bool)  [unwired: 7 in, 1 out]
        n240 = Array Subset(array="Command Params", length (row)=w380) -> (w381:string[][])  [unwired: 3 in]
        n241 = Select(t="Executing" ("Cmd Status"), s=w379, f="" ("Cmd Status")) -> (s? t:f=→"Cmd Status":string)
      }
      event "Command Selection": Double Click {
        n242 = event-data() -> ("Row"=w394:i32)  [unwired: 1 in]
        n243 = property on="Command Selection" class="MCListbox (strict)"() -> ("ItemNames"=w397:string[][])  [unwired: 2 in, 2 out]
        n244 = local read "Command Params"() -> (w393:string[][])
        n245 = Index Array(array=w397, index (row)=w394, index (col)=0) -> (element=w395:string)
        n246 = call <vilib>:"Invoke Commands.vi"("Command Params"=w393, "Function Name"=w395) -> ("Params"=w392:u8, "Started"=w387:bool)  [unwired: 7 in, 1 out]
        n247 = Array Subset(array=w393, length (row)=w392) -> (w391:string[][])  [unwired: 3 in]
        n248 = Select(t="Executing" ("Cmd Status"), s=w387, f="" ("Cmd Status")) -> (s? t:f=w388:string)
        n249 = local write "Cmd Status"(w388) -> ()
      }
      event "CheckList": Double Click {
        # "Shift clears all"
        # "Update symbols on the listbox"
        n250 = event-data() -> ("PlatMods.Shift"=w399:bool, "Row"=w401:i32)  [unwired: 1 in]
        n251 = case shown="True" w399 {
          tunnel: w401 -> [w405 _]
          tunnel: 1 -> [w404 _]
          frame False {
            n252 = property on="CheckList" class="LstBox (strict)"() -> ("Item Symbols"=w403:i32[])  [unwired: 2 in, 2 out]
            n253 = Replace Array Subset(array=w403, new element=w404, index=w405) -> (w402:i32[])
            n254 = property on="CheckList" class="LstBox (strict)"("Item Symbols"=w402) -> ()  [unwired: 2 in, 2 out]
          }
          frame True {
            w406 = 0 ("Top Row")
            n255 = property on="CheckList" class="LstBox (strict)"() -> ("Number of Rows"=w408:u32)  [unwired: 2 in, 2 out]
            n256 = Initialize Array(0, w408) -> (w407:i32[])
            n257 = property on="CheckList" class="LstBox (strict)"("Top Row"=w406, "Value"=w406, "Item Symbols"=w407) -> ()  [unwired: 2 in, 2 out]
          }
        }
      }
      event "CheckList": Key Down {
        # "Update symbols on the listbox\nLeft and right keys check and uncheck"
        n258 = event-data() -> ("VKey"=w412:T19)  [unwired: 1 in]
        n259 = case shown="\"Left\", \"Right\"" w412 {
          selector: w412 -> [w417 _]
          tunnel: eventvkey."Left" ("VKey") -> [w415 _]
          frame "Left", "Right" {
            n260 = Equal?(x=w415, y=w417) -> (x = y?=w416:bool)
            n261 = Select(t=0, s=w416, f=1) -> (s? t:f=w418:i32)
            n262 = property on="CheckList" class="LstBox (strict)"() -> ("Item Symbols"=w421:i32[])  [unwired: 2 in, 2 out]
            n263 = Replace Array Subset(array=w421, new element=w418, index="CheckList") -> (w420:i32[])
            n264 = property on="CheckList" class="LstBox (strict)"("Item Symbols"=w420) -> ()  [unwired: 2 in, 2 out]
          }
          frame Default {
          }
        }
      }
      event "Motor.Enable": Value Change {
        # "When the test mode otor enable helper is set, update that\ntree row item's value"
        n265 = event-data() -> ("NewVal"=w427:bool)  [unwired: 1 in]
        n266 = Unbundle("Motor") -> ("Value"=w426:dbl)  [unwired: 1 out]
        n267 = Select(t=w426, s=w427, f=0.0) -> (s? t:f=w424:dbl)
        n268 = call <vilib>:"NT Write Number.vi"("Numeric"=w424, "Name"=w423) -> ()  [unwired: 9 in, 1 out]
      }
      event "Test Slider": Value Change {
        # "When the test mode slider helper is set, update that\ntree row item's value"
        n269 = event-data() -> ("NewVal"=w430:dbl)  [unwired: 1 in]
        n270 = call <vilib>:"NT Write Number.vi"("Numeric"=w430, "Name"=w431) -> ()  [unwired: 9 in, 1 out]
      }
      event "On/Off": Value Change {
        # "When the test mode on/off helper value is set, update that\ntree row item's value"
        n271 = event-data() -> ("NewVal"=w435:bool)  [unwired: 1 in]
        n272 = Boolean To (0,1)(Boolean=w435) -> (0, 1=w434:i16)
        n273 = call <vilib>:"NT Write Number.vi"("Numeric"=w434, "Name"=w433) -> ()  [unwired: 9 in, 1 out]
      }
      event "Rev/Fwd": Value Change {
        # "When the test mode helper value for relays is set, update that\ntree row item's value"
        n274 = event-data() -> ("NewVal.Forward"=w443:bool, "NewVal.Reverse"=w442:bool)  [unwired: 1 in]
        n275 = Boolean To (0,1)(Boolean=w443) -> (0, 1=w439:i16)
        n276 = Boolean To (0,1)(Boolean=w442) -> (0, 1=w441:i16)
        n277 = Negate(x=w441) -> (-x=w440:i16)
        n278 = Add(x=w439, y=w440) -> (x+y=w438:i16)
        n279 = call <vilib>:"NT Write Number.vi"("Numeric"=w438, "Name"=w437) -> ()  [unwired: 9 in, 1 out]
      }
      event "Test Ring": Value Change {
        # "When a test mode helper value is selected from the ring,\nset the tree item's variable to the string value"
        n280 = event-data() -> ("NewVal"=w447:u16)  [unwired: 1 in]
        n281 = property on="Test Ring" class="Ring (strict)"() -> ("Strings []"=w448:string[])  [unwired: 2 in, 2 out]
        n282 = Index Array(array=w448, index=w447) -> (element=w446:string)
        n283 = call <vilib>:"NT Write String.vi"("String"=w446, "Name"=w445) -> ()  [unwired: 9 in, 1 out]
      }
      event "Rec Mode": Value Change {
        # "Update globals for recording mode and path to read log from.\nClear when logging and let NetworkTables set path for vision to\nuse."
        n284 = event-data() -> ("NewVal"=w459:enum32{"Stop", "Record", "Playback"})  [unwired: 1 in]
        n285 = global write "WPI_DashboardLogging Global.vi" "Logging Filename"(path "") -> ()
        n286 = global write "WPI_DashboardLogging Global.vi" "Recording"(w459) -> ()
        n287 = case shown="\"Playback\"" w459 {
          tunnel: w458 -> [_ w461 w470]
          tunnel: [_ _ w469] -> w456
          tunnel: [_ _ w468] -> _
          tunnel: w454 -> [_ _ w466]
          tunnel: cluster{i32, i32} {-250, 170} -> [_ _ w465]
          tunnel: [_ _ T20 {"Image Size"=TRUE, "Image Type"=TRUE, "Pixel Value"=TRUE, "ROI Information"=TRUE, "Zoom Factor"=FALSE} ("Image Information Shown:All Elements")] -> w452
          tunnel: [_ _ TRUE ("Zoom Factor")] -> w451
          tunnel: w450 -> [_ _ w462]
          frame Default {
          }
          frame "Stop", "Record" {
            # "Place Window too"
            n288 = invoke class="VI" method="FP.Close"(reference=w461) -> (reference out=w460:refnum<vi>)  [unwired: 2 in, 2 out]
            n289 = invoke class="VI" method="Abort VI"(reference=w460) -> ()  [unwired: 2 in, 3 out]
          }
          frame "Playback" {
            n290 = call "Open Playback Panel.vi"("Offset"=w465, "DB VI Ref"=w466, "Playback in"=w470) -> ("Playback out"=w467:refnum<vi>)  [unwired: 8 in]
            n291 = register-events(w467, w462) -> (reference out=w469:refnum<event-registration>, error out=w468:errorcluster)  [unwired: 2 in]
          }
        }
        n292 = property on="Camera Image" class="ImageControl"("Image Information Shown"=w452, "Image Information Visible"=w451) -> ()  [unwired: 2 in, 2 out]
        n293 = call <vilib>:"WPI_DashboardNT Log FieldName Cache.vi"("Operation"=enum16{"Lookup/Add", "Index", "Clear"}."Clear") -> ()  [unwired: 8 in, 3 out]
      }
      event Panel Close {
        w472 = enum32{"Stop", "Record", "Playback"}."Stop" ("Rec Mode")
        # "Playback window has been closed, abort"
        n294 = event-data() -> ()  [unwired: 1 in, 4 out]
        n295 = local write "Rec Mode"(w472) -> ()
        n296 = global write "WPI_DashboardLogging Global.vi" "Recording"(w472) -> ()
      }
      event Panel Close {
        # "Abort playback window and ourself"
        n297 = event-data() -> ()  [unwired: 1 in, 4 out]
        n298 = invoke class="VI" method="FP.Close"(reference=w476) -> (reference out=w475:refnum<vi>)  [unwired: 2 in, 2 out]
        n299 = invoke class="VI" method="Abort VI"(reference=w475) -> (error out=w474:errorcluster)  [unwired: 2 in, 2 out]
        n300 = invoke class="VI" method="Abort VI"(error in=w474) -> ()  [unwired: 2 in, 3 out]
      }
      event User Event {
        n301 = event-data() -> ("IDs"=w483:cluster{"RPC field ID":u16, "Unique ID":u16}, "String"=w482:string)  [unwired: 1 in]
        n302 = Bundle("IDs"=w483, "String"=w482) -> (w481:T8)  [unwired: 1 in]
        n303 = call <vilib>:"Retrieve RPC Response.vi"("RPC Response"=w481) -> ("Output"=w479:string[][])  [unwired: 10 in]
        n304 = Build Array (concatenate)(w477, w479) -> (w478:string[][])
        n305 = local write "Command Params"(w478) -> ()
        n306 = local write "Cmd Status"("" ("Cmd Status")) -> ()
      }
      event "Tree": Double Click {
        n307 = event-data() -> ("PlatMods"=w487:T23, "Tag"=w486:string)  [unwired: 1 in]
        n308 = Unbundle(w487) -> ("Shift"=w485:bool)  [unwired: 4 out]
        n309 = Not(x=w485) -> (.not. x?=w484:bool)
        n310 = call <vilib>:"NT Update Persistence.vi"("Persistence"=w484, "Name"=w486) -> ()  [unwired: 9 in, 1 out]
      }
    }
  }
  n311 = while {
    tunnel: w74 -> [w490]
    i -> [w493]
    stop <- FALSE stop-if-true
    n312 = Wait (ms)(milliseconds to wait=u32 100) -> ()  [unwired: 1 out]
    n313 = case shown="\"Playback\"" "Rec Mode" {
      tunnel: w493 -> [_ _ w508]
      tunnel: [u32 2829099 ("Base Color") u32 11141120 ("Target Color") w497] -> w489
      frame "Stop", Default {
        # "Reset the color, extra updates don't cost much"
      }
      frame "Record" {
      }
      frame "Playback" {
        # "Playback"
        n314 = Quotient & Remainder(x=w508, y=u32 50 ("milliseconds to wait")) -> (x-y*floor(x/y)=w504:u32)  [unwired: 1 out]
        n315 = Divide(x=w504, y=u32 50 ("milliseconds to wait")) -> (x/y=w501:dbl)
        n316 = Multiply(x=6.283185307179586, y=w501) -> (x*y=w506:dbl)
        n317 = Sine(x=w506) -> (sin(x)=w505:dbl)
        n318 = Absolute Value(x=w505) -> (abs(x)=w498:dbl)
        n319 = call "Interpolate RGB Color.vi"("Proportion"=w498, "Target Color"=u32 30976, "Base Color"=u32 2829099) -> ("Result Color"=w497:u32)  [unwired: 8 in]
      }
    }
    n320 = property class="Pane"(reference=w490, "PaneColor"=w489) -> ()  [unwired: 1 in, 2 out]
  }
  n321 = local write "Dashboard Tab"(T2."Drive" ("Dashboard Tab")) -> ()
  n322 = property on="On/Off" class="Bool (strict)"("Visible"=w45) -> ()  [unwired: 2 in, 2 out]
  n323 = property on="Motor" class="Clust (strict)"("Visible"=w45) -> ()  [unwired: 2 in, 2 out]
  n324 = property on="Progress" class="Clust (strict)"("Visible"=w45) -> ()  [unwired: 2 in, 2 out]
  n325 = property on="Test Ring" class="Ring (strict)"("Visible"=w45) -> ()  [unwired: 2 in, 2 out]
  n326 = property on="Rev/Fwd" class="Clust (strict)"("Visible"=w45) -> ()  [unwired: 2 in, 2 out]
  n327 = call-poly <vilib>:"NT Read Value.vi"("Name"="ZAcc") -> ("Numeric"=→"Z Acceleration":dbl)  [unwired: 9 in, 1 out]
  n328 = call-poly <vilib>:"NT Read Value.vi"("Name"="YAcc") -> ("Numeric"=→"Y Acceleration":dbl)  [unwired: 9 in, 1 out]
  n329 = while {
    tunnel: u16 1741 ("timeout ms (25000)") -> [w510]
    stop <- FALSE stop-if-true
    n330 = TCP Create Listener(10:w510) -> (0:w509:errorcluster, 3:w511:refnum<k5>)  [unwired: 4 in, 1 out]
    n331 = case shown="No Error" w509 {
      selector: w509 -> [w513 _]
      tunnel: w511 -> [w514 _]
      frame No Error {
        n332 = while {
          tunnel: w514 -> [w517]
          tunnel: w513 -> [w516]
          stop <- FALSE stop-if-true
          n333 = TCP Wait On Listener(8:w516, 11:w517) -> (0:w518:errorcluster, 4:w519:refnum<k5>)  [unwired: 2 in, 3 out]
          n334 = local write "TCP"(w519) -> ()
          n335 = case shown="No Error" w518 {
            frame No Error {
            }
            frame Error {
              n336 = Wait (ms)(milliseconds to wait=u32 1000) -> ()  [unwired: 1 out]
            }
          }
        }
      }
      frame Error {
        n337 = Wait (ms)(milliseconds to wait=u32 1000) -> ()  [unwired: 1 out]
      }
    }
  }
  n338 = call-poly <vilib>:"NT Read Value.vi"("Name"="XAcc") -> ("Numeric"=→"X Acceleration":dbl)  [unwired: 9 in, 1 out]
  n339 = local write "Command Selection"(u16 0 ("milliseconds to wait")) -> ()
  n340 = local write "Command Params"(string[][] [] ("Command Params")) -> ()
  n341 = global write "WPI_DashboardLogging Global.vi" "Recording"(w68) -> ()
  n342 = local write "Rec Mode"(w68) -> ()
  n343 = call <vilib>:"NT Write String.vi"("String"="Select Auto", "Name"="Auto Selector") -> ()  [unwired: 9 in, 1 out]
  n344 = call-poly <vilib>:"NT Read Value.vi"("Name"="Sonar") -> ("Numeric"=→"distance":dbl)  [unwired: 9 in, 1 out]
  n345 = call-poly <vilib>:"NT Write Value.vi"("Numeric"="Scaling factor (V/in)", "Name"="Scaling") -> ()  [unwired: 9 in, 1 out]
